vi "Bai3_6_C1.vi"() -> ()   [LabVIEW 2023]
panel:
  in  "Device Name":tag="Dev8"
  in  "Lines to Write":u16(ring) items=["0 - 7", "8 - 15", "16 - 23"]
  in  "Stop":bool=TRUE
  in  "error in":errorcluster
  out "error out":errorcluster
  in  "stop":bool
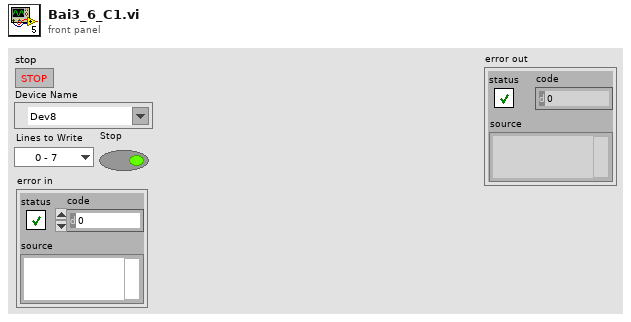
[diagram p1: front panel]
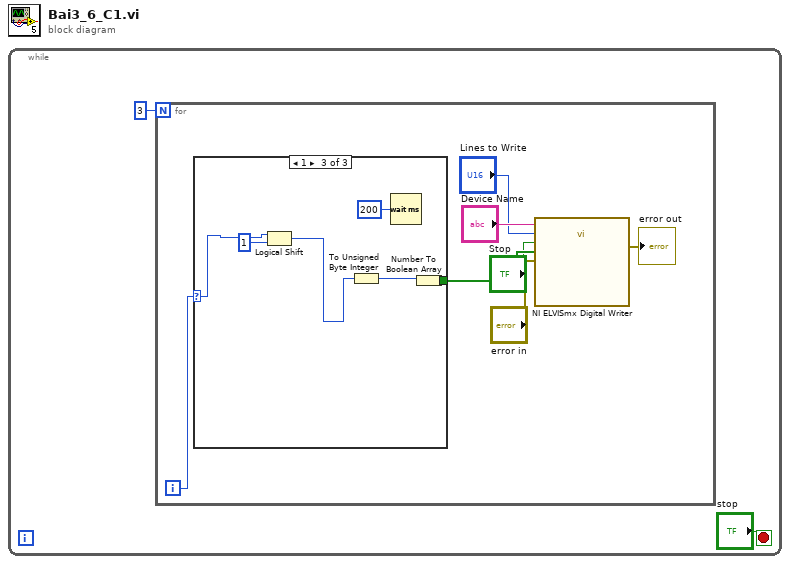
[diagram p0: block diagram]
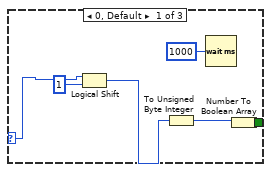
[diagram p2: hidden frame]
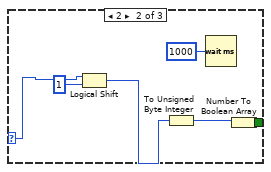
[diagram p3: hidden frame]
diagram:
  n1 = while {
    stop <- "stop" stop-if-true
    n2 = for {
      N: 3 -> [_]
      i -> [w3]
      n3 = case shown="1" w3 {
        selector: w3 -> [w10 w16 w22]
        tunnel: [w13 w19 w25] -> w9
        frame 0, Default {
          n4 = Logical Shift(y=w10, x=1) -> (x << y=w15:i32)
          n5 = To Unsigned Byte Integer(number=w15) -> (unsigned 8bit integer=w14:u8)
          n6 = Wait (ms)(milliseconds to wait=u32 1000) -> ()  [unwired: 1 out]
          n7 = Number To Boolean Array(number=w14) -> (Boolean array=w13:bool[])
        }
        frame 2 {
          n8 = Logical Shift(y=w16, x=1) -> (x << y=w21:i32)
          n9 = To Unsigned Byte Integer(number=w21) -> (unsigned 8bit integer=w20:u8)
          n10 = Wait (ms)(milliseconds to wait=u32 1000) -> ()  [unwired: 1 out]
          n11 = Number To Boolean Array(number=w20) -> (Boolean array=w19:bool[])
        }
        frame 1 {
          n12 = Logical Shift(y=w22, x=1) -> (x << y=w27:i32)
          n13 = To Unsigned Byte Integer(number=w27) -> (unsigned 8bit integer=w26:u8)
          n14 = Wait (ms)(milliseconds to wait=u32 200) -> ()  [unwired: 1 out]
          n15 = Number To Boolean Array(number=w26) -> (Boolean array=w25:bool[])
        }
      }
      n16 = call "NI ELVISmx Digital Writer"("Device Name"="Device Name", "Lines to Write"="Lines to Write", "Stop"="Stop", "DO Lines"=w9, "error in"="error in") -> ("error out"=→"error out":errorcluster)  [unwired: 14 in]
    }
  }
